vi "testAddStatesToQueueEolHandling3.vi"(8 "error in (no error)":errorcluster, 11 "testStateMachineUtilities in":refnum<class "testStateMachineUtilities.lvclass">=refnum) -> (0 "error out":errorcluster, 3 "testStateMachineUtilities out":refnum<class "testStateMachineUtilities.lvclass">)   [LabVIEW 2016, in "testStateMachineUtilities.lvclass"]
uses:
  testStateMachineUtilities.lvclass
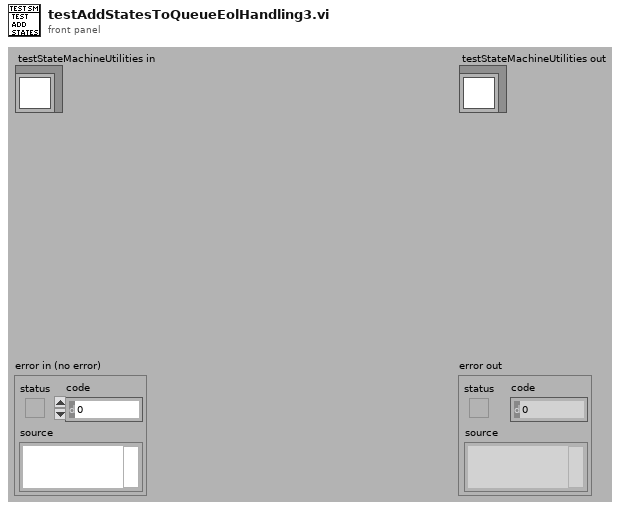
[diagram p1: front panel]
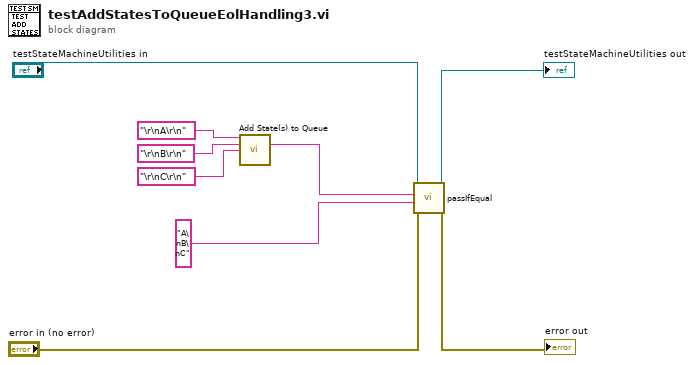
[diagram p0: block diagram]
diagram:
  n1 = call "Add State(s) to Queue.vi"("State(s) in Front (\"\")"="\r\nA\r\n" ("State(s) in Front"), "State(s) in (\"\")"="\r\nB\r\n" ("State(s) in Front"), "State(s) at Back (\"\")"="\r\nC\r\n" ("State(s) in Front")) -> ("States Out"=w7:string)  [unwired: 12 in]
  n2 = call-dynamic "passIfEqual.vi"("error in (no error)"="error in (no error)", "y"="A\nB\nC" ("State(s) at Back"), "x"=w7, "TestCase in"="testStateMachineUtilities in") -> ("error out"=→"error out":errorcluster, "TestCase out"=→"testStateMachineUtilities out":refnum<class "testStateMachineUtilities.lvclass">)  [unwired: 6 in]
